vi "_Obsolete_PathPlanner_TrajectoryWaypoint_New_Empty.vi"() -> (3 "PathPlannerWaypoint":T1={"AnchorPoint"={"X"=0.0, "Y"=0.0}, "PrevControl"={"X"=0.0, "Y"=0.0}, "NextControl"={"X"=0.0, "Y"=0.0}, "HolonomicRotation"={"VALUE"=0.0, "COS"=1.0, "SIN"=0.0}, "VelOverride"=0.0, "isReversal"=FALSE} {"HolonomicRotation"."SIN" format="%13.4f"; "HolonomicRotation"."COS" format="%13.4f"; "HolonomicRotation"."VALUE" format="%13.4f"; "NextControl"."Y" format="%14.3f"; "NextControl"."X" format="%14.3f"; "PrevControl"."Y" format="%14.3f"; "PrevControl"."X" format="%14.3f"; "AnchorPoint"."Y" format="%14.3f"; "AnchorPoint"."X" format="%14.3f"})   [LabVIEW 2019, in "PathPlanner24.lvlib"]
uses:
  PathPlanner24.lvlib
  TypeDef/PathPlannerWaypoint.ctl
  <vilib>/Rock Robotics/WPI/ThirdParty/JAS_Junk/TrajLib/TypeDef/TRANSLATION2D.ctl
  <vilib>/Rock Robotics/WPI/ThirdParty/JAS_Junk/TrajLib/TypeDef/ROTATION2D.ctl
  <vilib>/Rock Robotics/WPI/ThirdParty/JAS_Junk/TrajLib/Trajectory_Library.lvlib
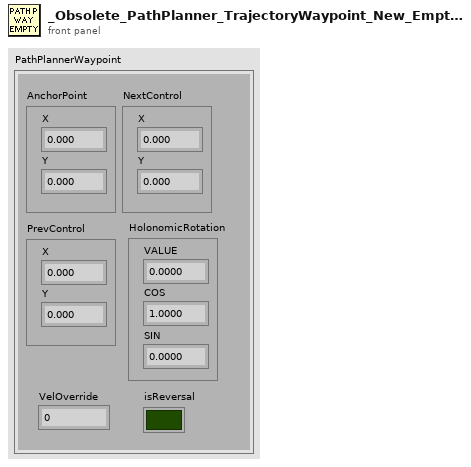
[diagram p1: front panel]
types:
  T1 = typedef "PathPlanner24.lvlib/PathPlannerWaypoint.ctl" = cluster{"AnchorPoint":T2, "PrevControl":T2, "NextControl":T2, "HolonomicRotation":T3, "VelOverride":dbl, "isReversal":bool}
  T2 = typedef "Trajectory_Library.lvlib/TRANSLATION2D.ctl" = cluster{"X":dbl, "Y":dbl}
  T3 = typedef "Trajectory_Library.lvlib/ROTATION2D.ctl" = cluster{"VALUE":dbl, "COS":dbl, "SIN":dbl}
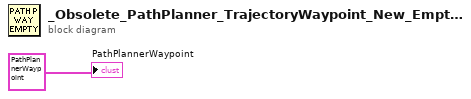
[diagram p0: block diagram]
diagram:
  "PathPlannerWaypoint" <- T1 {"AnchorPoint"={"X"=0.0, "Y"=0.0}, "PrevControl"={"X"=0.0, "Y"=0.0}, "NextControl"={"X"=0.0, "Y"=0.0}, "HolonomicRotation"={"VALUE"=0.0, "COS"=1.0, "SIN"=0.0}, "VelOverride"=0.0, "isReversal"=FALSE} ("PathPlannerWaypoint")
